vi "Draw_single_Box.vi"(0 "Picture in":picture, 1 "color(black)":u32(colorbox)=16777217, 5 "mm Per Pixel":dbl format="%.2f", 7 "Min Values":dbl[](array[numeric]) format="%.2f", 9 "Box Coordinates":cluster{"Max":dbl, "Min":dbl}[](array[cluster])=[{"Max"=16000.0, "Min"=14000.0}, {"Max"=1000.0, "Min"=-1000.0}, {"Max"=700.0, "Min"=0.0}] {"Min" format="%.1f"; "Max" format="%.1f"}, 11 "View":T1, 12 "Pixels per Axis":i16[](array[numeric]), 13 "fill?(F)":bool) -> (4 "Picture out":picture)   [LabVIEW 2010]
uses:
  Pict_Plot_Axis.ctl
  Axis.ctl
panel:
  # "X                Y               Z"
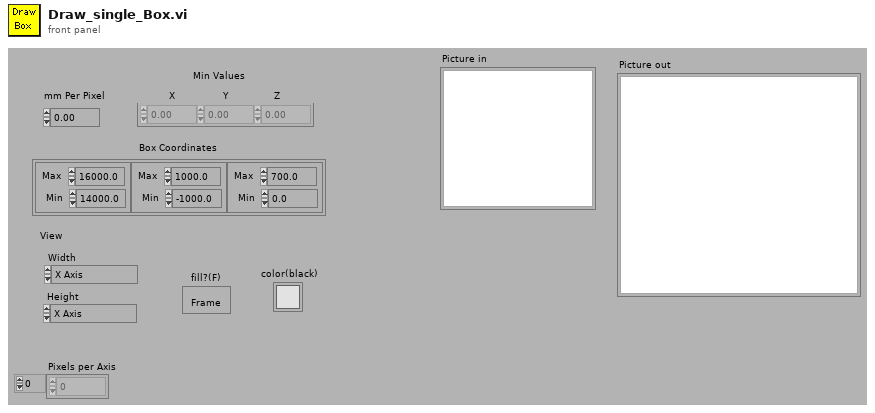
[diagram p1: front panel]
types:
  T1 = typedef "Pict_Plot_Axis.ctl" = cluster{"Width":T2, "Height":T2}
  T2 = typedef "Axis.ctl" = enum16{"X Axis", "X Axis -ve", "Y Axis", "Y Axis -ve", "Z Axis", "Z Axis -ve"}
  T3 = cluster{"left":i16, "top":i16, "right":i16, "bottom":i16}
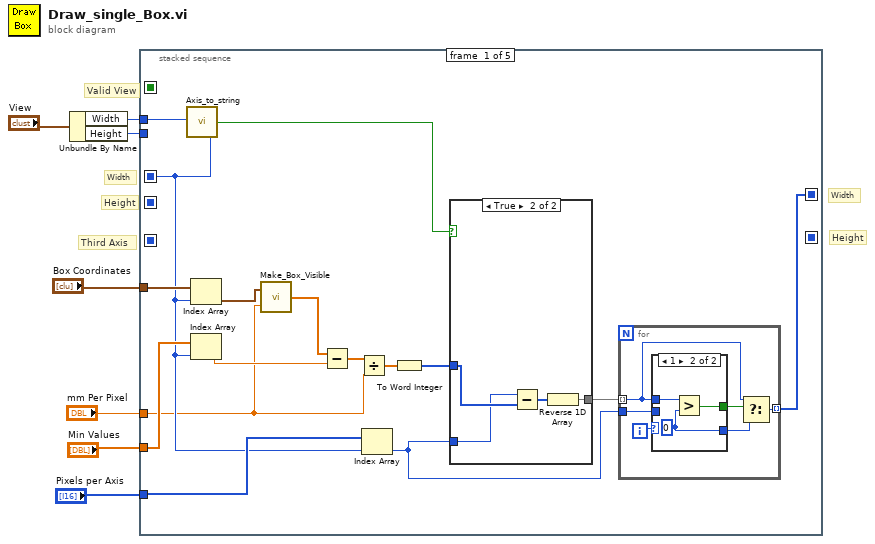
[diagram p0: block diagram]
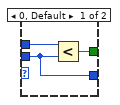
[diagram p2: hidden frame]
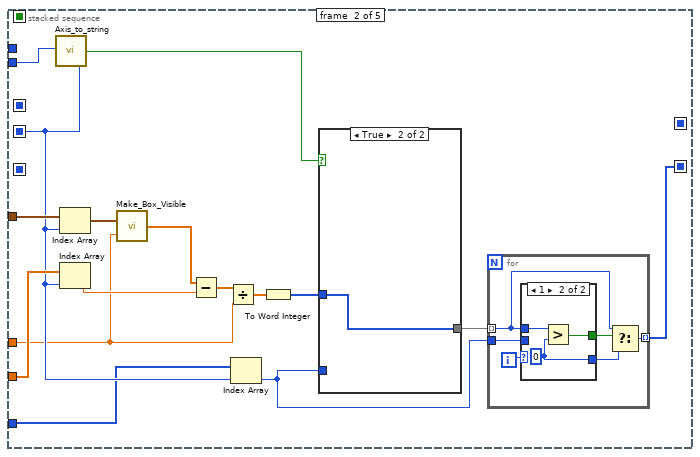
[diagram p4: hidden frame]
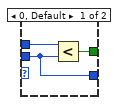
[diagram p5: hidden frame]
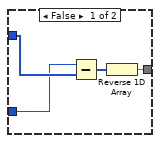
[diagram p6: hidden frame]
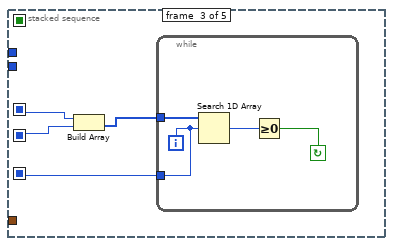
[diagram p7: hidden frame]
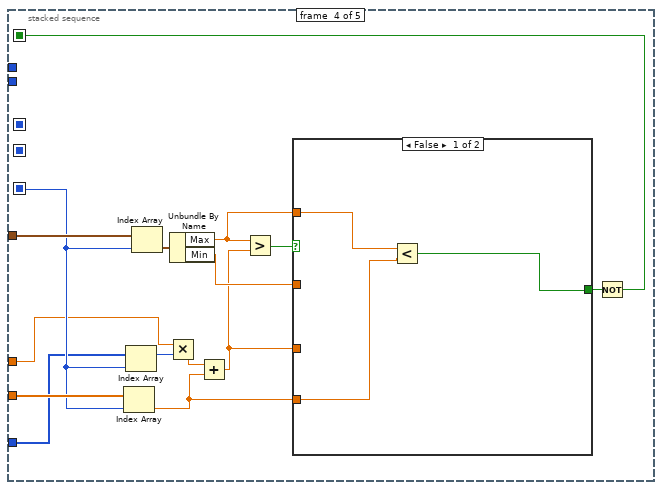
[diagram p8: hidden frame]
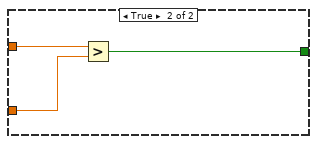
[diagram p9: hidden frame]
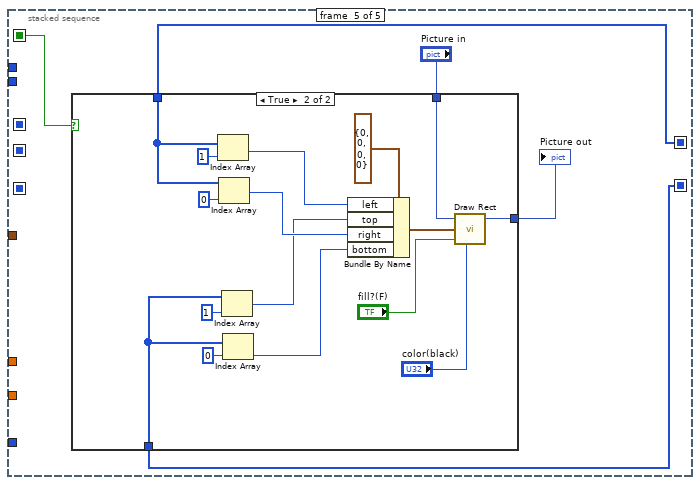
[diagram p10: hidden frame]
diagram:
  # "Height"
  # "Width"
  # "Valid View"
  # "Third Axis"
  # "Height"
  # "Width"
  n1 = Unbundle By Name("View") -> ("Width"=w3:T2, "Height"=w2:T2)
  n2 = stacked-sequence {
    seq-local: [w11 _ _ _ _] -> [_ _ _ _ w107]
    seq-local: [_ w42 _ _ _] -> [_ _ _ _ w106]
    seq-local: [_ w46 _ _ _] -> [_ _ w76 _ _]
    seq-local: [w13 _ _ _ _] -> [_ _ w77 _ _]
    seq-local: [_ _ w74 _ _] -> [_ _ _ w93 _]
    seq-local: [_ _ _ w86 _] -> [_ _ _ _ w103]
    tunnel: "Box Coordinates" -> [w23 w56 _ w95 _]
    tunnel: "Min Values" -> [w22 w54 _ w94 _]
    tunnel: "mm Per Pixel" -> [w9 w41 _ w90 _]
    tunnel: w3 -> [w12 _ _ _ _]
    tunnel: w2 -> [_ w47 _ _ _]
    tunnel: "Pixels per Axis" -> [w16 w45 _ w92 _]
    frame #0 {
      n3 = call "Axis_to_string.vi"("Axis"=w12) -> ("Reverse Scale"=w19:bool, "Index"=w13:i32)  [unwired: 1 out]
      n4 = Index Array(array=w23, index=w13) -> (element=w10:cluster{"Max":dbl, "Min":dbl})
      n5 = Index Array(array=w22, index=w13) -> (element=w20:dbl)
      n6 = call "Make_Box_Visible.vi"("mm Per Pixel"=w9, "X"=w10) -> ("Array"=w8:dbl[])
      n7 = Subtract(x=w8, y=w20) -> (x-y=w21:dbl[])
      n8 = Divide(x=w21, y=w9) -> (x/y=w18:dbl[])
      n9 = Index Array(array=w16, index=w13) -> (element=w14:i16)
      n10 = To Word Integer(number=w18) -> (16bit integer=w17:i16[])
      n11 = case shown="True" w19 {
        tunnel: w17 -> [w36 w40]
        tunnel: [w36 w38] -> w15
        tunnel: w14 -> [_ w37]
        frame False {
        }
        frame True {
          n12 = Subtract(x=w37, y=w40) -> (x-y=w39:i16[])
          n13 = Reverse 1D Array(array=w39) -> (reversed array=w38:i16[])
        }
      }
      n14 = for {
        tunnel: w15 -> [w26] mode=indexing
        tunnel: w14 -> [w28]
        tunnel: [w24] -> w11 mode=indexing
        i -> [w29]
        n15 = case shown="1" w29 {
          tunnel: w26 -> [w32 w35]
          tunnel: w28 -> [w30 _]
          tunnel: [w31 w34] -> w27
          tunnel: [w30 w33] -> w25
          frame 0, Default {
            n16 = Less?(x=w32, y=w30) -> (x < y?=w31:bool)
          }
          frame 1 {
            w33 = i16 0 ("y")
            n17 = Greater?(x=w35, y=w33) -> (0:w34:bool)
          }
        }
        n18 = Select(t=w26, s=w27, f=w25) -> (s? t:f=w24:i16)
      }
    }
    frame #1 {
      n19 = call "Axis_to_string.vi"("Axis"=w47) -> ("Reverse Scale"=w50:bool, "Index"=w46:i32)  [unwired: 1 out]
      n20 = Index Array(array=w56, index=w46) -> (element=w55:cluster{"Max":dbl, "Min":dbl})
      n21 = Index Array(array=w54, index=w46) -> (element=w52:dbl)
      n22 = call "Make_Box_Visible.vi"("mm Per Pixel"=w41, "X"=w55) -> ("Array"=w51:dbl[])
      n23 = Subtract(x=w51, y=w52) -> (x-y=w53:dbl[])
      n24 = Divide(x=w53, y=w41) -> (x/y=w49:dbl[])
      n25 = Index Array(array=w45, index=w46) -> (element=w43:i16)
      n26 = To Word Integer(number=w49) -> (16bit integer=w48:i16[])
      n27 = case shown="True" w50 {
        tunnel: w48 -> [w72 w73]
        tunnel: [w70 w73] -> w44
        tunnel: w43 -> [w69 _]
        frame False {
          n28 = Subtract(x=w69, y=w72) -> (x-y=w71:i16[])
          n29 = Reverse 1D Array(array=w71) -> (reversed array=w70:i16[])
        }
        frame True {
        }
      }
      n30 = for {
        tunnel: w44 -> [w59] mode=indexing
        tunnel: w43 -> [w61]
        tunnel: [w57] -> w42 mode=indexing
        i -> [w62]
        n31 = case shown="1" w62 {
          tunnel: w59 -> [w65 w68]
          tunnel: w61 -> [w63 _]
          tunnel: [w64 w67] -> w60
          tunnel: [w63 w66] -> w58
          frame 0, Default {
            n32 = Less?(x=w65, y=w63) -> (x < y?=w64:bool)
          }
          frame 1 {
            w66 = i16 0 ("y")
            n33 = Greater?(x=w68, y=w66) -> (0:w67:bool)
          }
        }
        n34 = Select(t=w59, s=w60, f=w58) -> (s? t:f=w57:i16)
      }
    }
    frame #2 {
      n35 = Build Array(w77, w76) -> (w75:i32[])
      n36 = while {
        tunnel: [w78] -> w74
        tunnel: w75 -> [w81]
        i -> [w78]
        stop <- w79 continue-if-true
        n37 = Search 1D Array(1D array=w81, element=w78) -> (index of element=w80:i32)  [unwired: 1 out]
        n38 = Greater Or Equal To 0?(x=w80) -> (x >= 0?=w79:bool)
      }
    }
    frame #3 {
      n39 = Index Array(array=w94, index=w93) -> (element=w83:dbl)
      n40 = Index Array(array=w92, index=w93) -> (element=w91:i16)
      n41 = Index Array(array=w95, index=w93) -> (element=w96:cluster{"Max":dbl, "Min":dbl})
      n42 = Multiply(x=w90, y=w91) -> (x*y=w84:dbl)
      n43 = Unbundle By Name(w96) -> ("Max"=w85:dbl, "Min"=w88:dbl)
      n44 = Add(x=w84, y=w83) -> (x+y=w82:dbl)
      n45 = Greater?(x=w85, y=w82) -> (0:w89:bool)
      n46 = case shown="False" w89 {
        tunnel: w88 -> [_ w102]
        tunnel: w82 -> [_ w101]
        tunnel: [w97 w100] -> w87
        tunnel: w85 -> [w99 _]
        tunnel: w83 -> [w98 _]
        frame False {
          n47 = Less?(x=w99, y=w98) -> (x < y?=w97:bool)
        }
        frame True {
          n48 = Greater?(x=w102, y=w101) -> (0:w100:bool)
        }
      }
      n49 = Not(x=w87) -> (.not. x?=w86:bool)
    }
    frame #4 {
      n50 = case shown="True" w103 {
        tunnel: w107 -> [_ w122]
        tunnel: w106 -> [_ w119]
        tunnel: "Picture in" -> [w108 w117]
        tunnel: [w108 w116] -> w104
        frame False {
        }
        frame True {
          n51 = Index Array(array=w122, index=1 ("Index")) -> (element=w112:i16)
          n52 = Index Array(array=w122, index=0 ("Index")) -> (element=w111:i16)
          n53 = Index Array(array=w119, index=1 ("Index")) -> (element=w110:i16)
          n54 = Index Array(array=w119, index=0 ("Index")) -> (element=w109:i16)
          n55 = Bundle By Name(cluster=T3 {"left"=0, "top"=0, "right"=0, "bottom"=0} ("rect"), "left"=w112, "top"=w110, "right"=w111, "bottom"=w109) -> (w115:T3)
          n56 = call <vilib>:"Draw Rect.vi"("picture"=w117, "rect"=w115, "fill?(F)"="fill?(F)", "color(black)"="color(black)") -> ("new picture"=w116:picture)  [unwired: 1 in, 4 out]
        }
      }
      "Picture out" <- w104
    }
  }
